vi "Write Report.vi"(8 "error in (no error)":errorcluster, 10 "Resource In":variant, 11 "Analyze Results Fluence in":refnum<class "Analyze Results Fluence.lvclass">) -> (0 "error out":errorcluster, 2 "Resource Out":variant, 3 "Analyze Results Fluence out":refnum<class "Analyze Results Fluence.lvclass">)   [LabVIEW 2014, in "Analyze Results Fluence.lvclass"]
uses:
  Analyze Results Fluence.lvclass
  <vilib>/Utility/config.llb/Config Data RefNum.ctl
  Results Base/Analyze Results Base.lvclass/Analyze Results Base.ctl
  Analyze Results Fluence.lvclass/Analyze Results Fluence.ctl
  Results Base/Read Section.vi
  <vilib>/Utility/config.llb/Write Key (Double).vi
  <vilib>/Utility/config.llb/Write Key (I32).vi
  <vilib>/Utility/config.llb/NI_LVConfig.lvlib
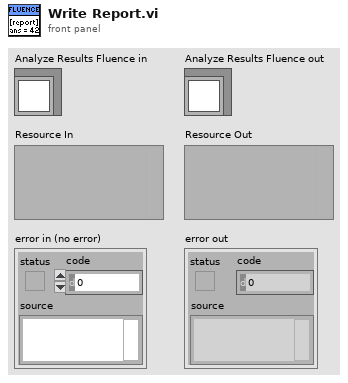
[diagram p1: front panel]
types:
  T1 = typedef "NI_LVConfig.lvlib/Config Data RefNum.ctl" = refnum<k1>
  T2 = typedef "Analyze.lvlib/Analyze Fluence.lvclass/Fluence Info.ctl" = cluster{"Fluence J/cm^2":dbl[unit], "Energy in Area":dbl[unit], "max value":i64, "Max fluence area":cluster{"Left":i32, "Top":i32, "Right":i32, "Bottom":i32}}
  T3 = cluster{"Left":i32, "Top":i32, "Right":i32, "Bottom":i32}
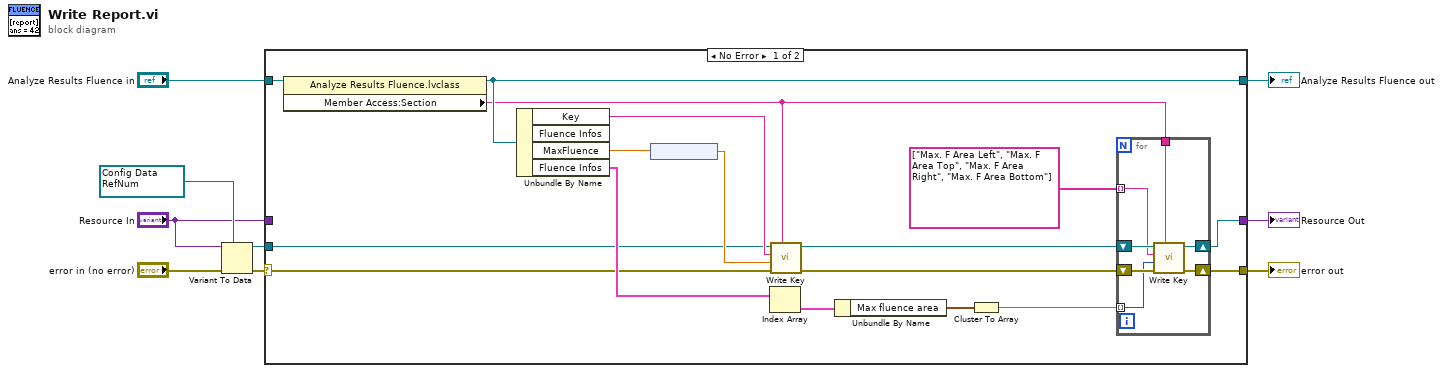
[diagram p0: block diagram]
diagram:
  w9 = T1 refnum items=["config data"] ("refnum")
  n1 = Variant To Data(error in="error in (no error)", type=w9, Variant="Resource In") -> (data=w8:T1, error out=w7:errorcluster)
  n2 = case shown="No Error" w7 {
    selector: w7 -> [w15 w35]
    tunnel: w8 -> [w16 _]
    tunnel: "Analyze Results Fluence in" -> [w26 w34]
    tunnel: [w25 w34] -> w3
    tunnel: [w12 w36] -> w2
    tunnel: [w11 w35] -> w1
    tunnel: "Resource In" -> [_ w36]
    frame No Error {
      n3 = property class="Analyze Results Fluence.lvclass"(reference=w26) -> (reference out=w25:refnum<class "Analyze Results Fluence.lvclass">, "Member Access:Section"=w13:string)  [unwired: 1 in, 1 out]
      n4 = Unbundle By Name(w25) -> ("Key"=w21:string, "MaxFluence"=w20:dbl[unit], "Fluence Infos"=w18:T2[])  [unwired: 1 out]
      n5 = node(w20) -> (w19:dbl)
      n6 = Index Array(array=w18) -> (element=w17:T2)  [unwired: 1 in]
      n7 = call-poly <vilib>:"Write Key.vi"("section"=w13, "error in (no error)"=w15, "value"=w19, "key"=w21, "refnum"=w16) -> ("error out"=w10:errorcluster, "refnum out"=w23:T1)  [unwired: 4 in, 1 out]
      n8 = Unbundle By Name(w17) -> ("Max fluence area"=w14:T3)
      n9 = Cluster To Array(cluster=w14) -> (array=w22:i32[])
      n10 = for {
        tunnel: w22 -> [w28] mode=indexing
        shift-right: [w32] -> w12
        shift-left: w23 -> [w33]
        tunnel: string[] ["Max. F Area Left", "Max. F Area Top", "Max. F Area Right", "Max. F Area Bottom"] -> [w31] mode=indexing
        shift-right: [w29] -> w11
        shift-left: w10 -> [w30]
        tunnel: w13 -> [w27]
        n11 = call-poly <vilib>:"Write Key.vi"("section"=w27, "error in (no error)"=w30, "value"=w28, "key"=w31, "refnum"=w33) -> ("error out"=w29:errorcluster, "refnum out"=w32:T1)  [unwired: 4 in, 1 out]
      }
    }
    frame Error {
    }
  }
  "error out" <- w1
  "Analyze Results Fluence out" <- w3
  "Resource Out" <- w2
